vi "Delayed Send to Consumer - Core.vi"(0 "Father of all uServices in":refnum<class "Father of all uServices.lvclass">, 5 "Seconds":dbl, 7 "Case ID":variant, 9 "Data":variant, 11 "error in (no error)":errorcluster) -> (4 "Father of all uServices out":refnum<class "Father of all uServices.lvclass">, 15 "error out":errorcluster)   [LabVIEW 2026, in "TALOS.lvlib" / "Father of all uServices.lvlib" / "Father of all uServices.lvclass"]
doc: "Core VI for sending a message to the consumer with a delay. The message will be enqueued in front of all existing messages"
uses:
  Father of all uServices.lvclass
  C:/LabVIEW Code/TALOS/builds/Actor Framework PPL/Actor Framework.lvlibp/1abvi3w/vi.lib/ActorFramework/Actor/Actor.lvclass
  Father of all uServices Messages/Consumer Msg/Consumer Msg.lvclass/Consumer Msg.ctl
  Ancestor/Ancestor/Ancestor.lvclass/Ancestor.ctl
  85e9c20f-20f1-49c0-91c7-221f83514489.vi
  Father of all uServices Messages/Consumer Msg/Send Consumer.vi
  Support VIs/Substitute Error.vi
  Support VIs/Generate Error.vi
  FGV/Error Memory/Get Error Description.vi
  Support VIs/Get PC name.vi
  Ancestor/Ancestor/Read ID.vi
  Support VIs/Get Class Name.vi
  FGV/Error Memory/Error Memory Core.vi
  <vilib>/AdvancedString/Delimited String to 1D String Array.vi
  <vilib>/AdvancedString/Delimited String to 1D String Array (string).vi
  Support VIs/Circus Root Path.vi
  FGV/Error Memory/Error Crt Lvl checker.vi
  FGV/Error Memory/Error Memory Core.vi/40c8088d-b597-4017-91af-faa98e00292e.vi
  FGV/Error Memory/Error Memory Core.vi/d4a3ab98-063c-4e44-b43d-fbdcfe6c2be2.vi
  builds/Actor Framework PPL/Actor Framework.lvlibp/1abvi3w/vi.lib/ActorFramework/Actor/Read Self Enqueuer.vi
  <userlib>/_OpenG.lib/lvdata/lvdata.llb/Get Strings from Enum__ogtk.vi
  builds/Actor Framework PPL/Actor Framework.lvlibp/1abvi3w/vi.lib/ActorFramework/Message Enqueuer/Enqueue.vi
  Support VIs/Global Memory.vi
  <vilib>/Utility/LVClass/Get LV Class Name.vi
  Support VIs/Is in Packed Library.vi
  Support VIs/TALOS Root path.vi
  Support VIs/Read CSV worksheet.vi
  Support VIs/Global Constants.vi
  <vilib>/Utility/error.llb/General Error Handler.vi
  Support VIs/Error Log.vi
  Father of all uServices Messages/Consumer Msg/Consumer Msg.lvclass
  Ancestor/Ancestor/Ancestor.lvclass
  <vilib>/Comparison/Equal/Equal Functor/Equal Functor.lvclass
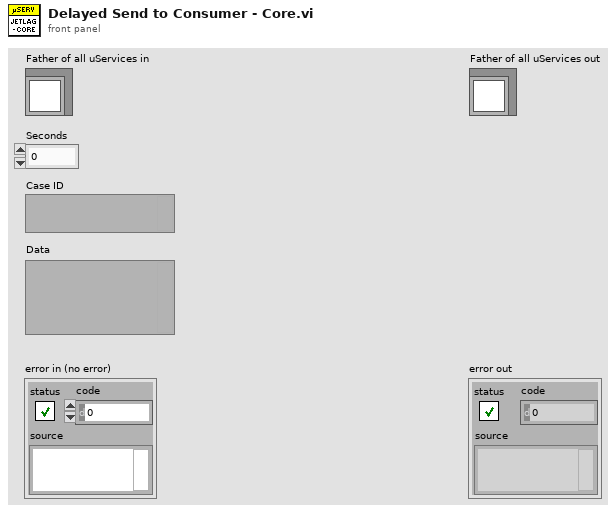
[diagram p1: front panel]
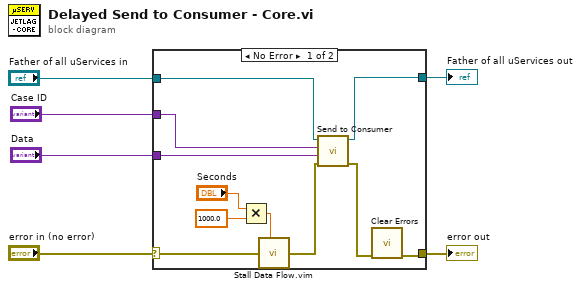
[diagram p0: block diagram]
diagram:
  n1 = case shown="No Error" "error in (no error)" {
    selector: "error in (no error)" -> [w15 w19]
    tunnel: [w7 w19] -> w5
    tunnel: [w16 w18] -> w3
    tunnel: "Father of all uServices in" -> [w17 w18]
    tunnel: "Data" -> [w10 _]
    tunnel: "Case ID" -> [w9 _]
    frame No Error {
      n2 = Multiply(x="Seconds", y=1000.0) -> (x*y=w13:dbl)
      n3 = call "Stall Data Flow.vim"("value in"=w15, "milliseconds to wait"=w13) -> ("value out"=w11:errorcluster)  [unwired: 1 out]
      n4 = call "Send to Consumer.vi"("error in (no error)"=w11, "Data"=w10, "Case ID"=w9, "uService Template in"=w17) -> ("error out"=w8:errorcluster, "uService Template out"=w16:refnum<class "Father of all uServices.lvclass">)  [unwired: 6 in]
      n5 = call <vilib>:"Clear Errors.vi"("error in (no error)"=w8) -> ("error out"=w7:errorcluster)  [unwired: 5 in, 1 out]
    }
    frame Error {
    }
  }
  "error out" <- w5
  "Father of all uServices out" <- w3
